vi "fissionReactorLogicAdapter.vi"(7 "Peripheral":string, 9 "State":T1={"Burn Rate"=0.0, "Formed"=FALSE, "Reactor Build Properties"={"Fuel Rods"=0, "Control Rods"=0, "Volume (m³)"=0, "Fuel Surface Area (m²)"=0, "Cooled Coolant Tank (mB)"=0, "Fuel Capacity (mB)"=0, "Heat Capacity (J/K)"=0.0, "Max Burn Rate"=0, "Max Heating Rate (mB/t)"=0, "Boil Efficiency"=0.0, "Coolant Type"=enum."Water", "Heated Coolant Tank (mB)"=0}, "Fission Reactor Build Specifications"={"Length (m)"=3, "Width (m)"=3, "Height (m)"=4, "Coolant Type"=enum."Water"}} {"Fission Reactor Build Specifications"."Height (m)" min=4 max=18 step=1; "Fission Reactor Build Specifications"."Width (m)" min=3 max=18 step=1; "Fission Reactor Build Specifications"."Length (m)" min=3 max=18 step=1; "Reactor Build Properties"."Boil Efficiency" format="%#.6g"}, 10 "Function":string, 11 "Mode":enum16{"Publish", "Read", "Handle", "Command"}(ring)) -> (3 "JSON":string)   [LabVIEW 2026]
uses:
  fissionReactor_State.ctl
  Fission Reactor Build Properties.ctl
  Fission Reactor Build Specifications.ctl
  Reactor Functions.ctl
  fissionReactor_Controls.ctl
  JSONBoolean.vi
  JSONInt64.vi
  JSONDouble.vi
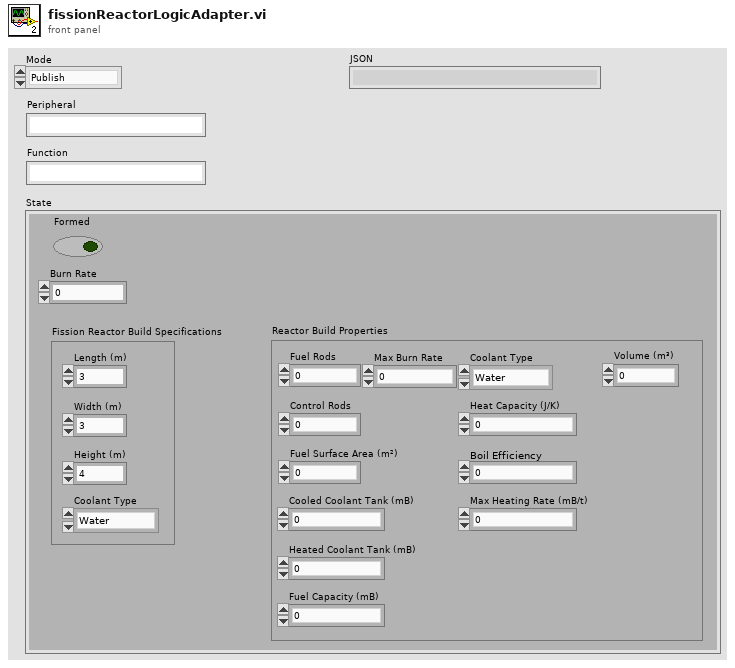
[diagram p1: front panel]
types:
  T1 = typedef "fissionReactor_State.ctl" = cluster{"Burn Rate":dbl, "Formed":bool, "Reactor Build Properties":T2, "Fission Reactor Build Specifications":T3}
  T2 = typedef "Fission Reactor Build Properties.ctl" = cluster{"Fuel Rods":i32, "Control Rods":i32, "Volume (m³)":i32, "Fuel Surface Area (m²)":i32, "Cooled Coolant Tank (mB)":i32, "Fuel Capacity (mB)":i64, "Heat Capacity (J/K)":dbl, "Max Burn Rate":i64, "Max Heating Rate (mB/t)":i64, "Boil Efficiency":dbl, "Coolant Type":enum16{"Water", "Sodium"}, "Heated Coolant Tank (mB)":i64}
  T3 = typedef "Fission Reactor Build Specifications.ctl" = cluster{"Length (m)":i32, "Width (m)":i32, "Height (m)":i32, "Coolant Type":enum16{"Water", "Sodium"}}
  T4 = typedef "fissionReactor_Controls.ctl" = cluster{"Burn Rate":dbl}
  T5 = typedef "Reactor Functions.ctl" = enum16{"isFormed", "getLength", "getWidth", "getHeight", "getMinPos", "getMaxPos", "activate", "getActualBurnRate", "getBoilEfficiency", "getBurnRate", "getCoolant", "getCoolantCapacity", "getCoolantFilledPercentage", "getCoolantNeeded", "getDamagePercent"}
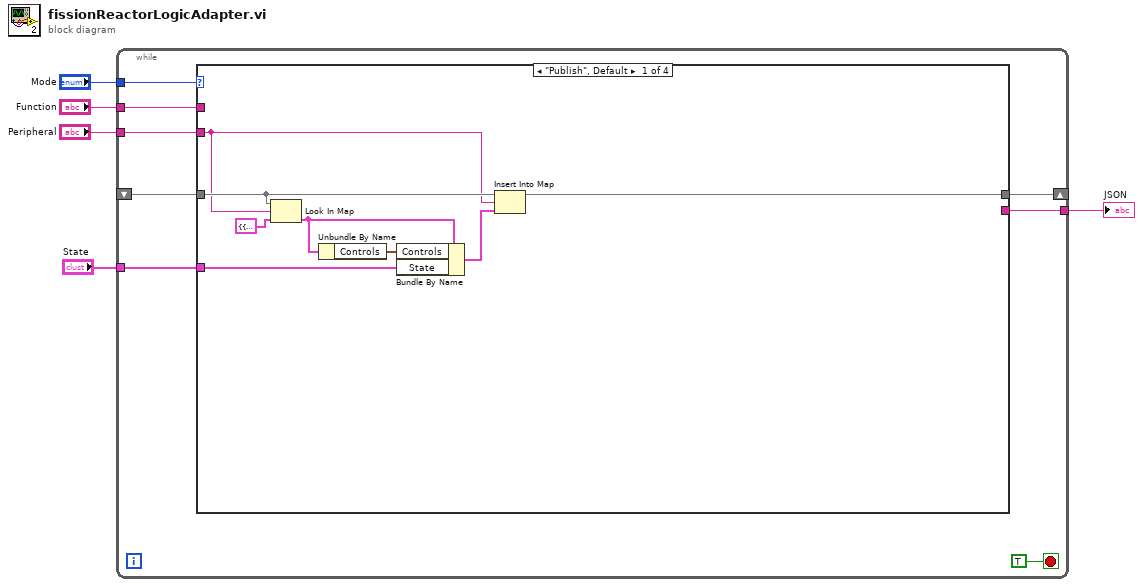
[diagram p0: block diagram]
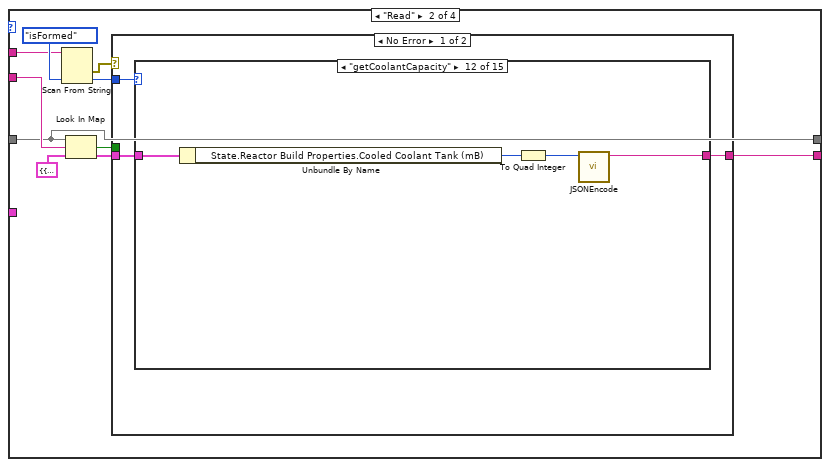
[diagram p2: hidden frame]
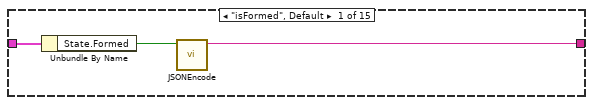
[diagram p3: hidden frame]
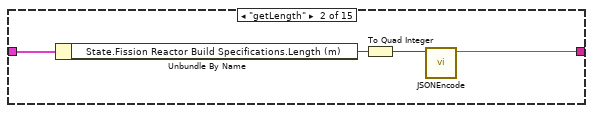
[diagram p4: hidden frame]
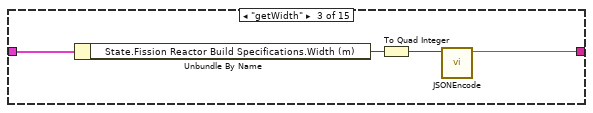
[diagram p5: hidden frame]
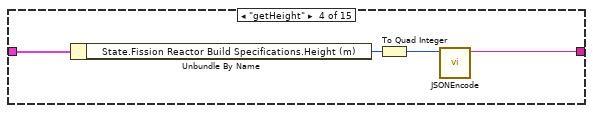
[diagram p6: hidden frame]
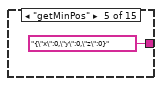
[diagram p7: hidden frame]
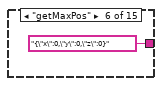
[diagram p8: hidden frame]
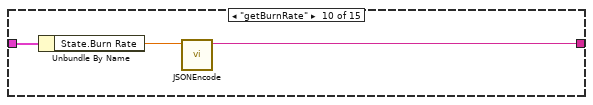
[diagram p12: hidden frame]
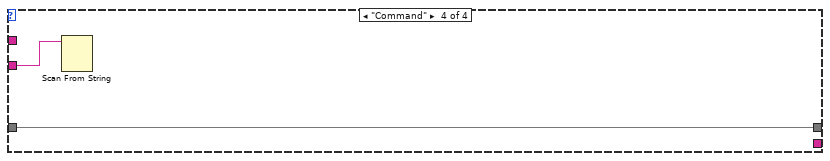
[diagram p19: hidden frame]
diagram:
  n1 = while {
    tunnel: "Mode" -> [w12]
    tunnel: "Peripheral" -> [w11]
    shift-right: [w8] -> _
    shift-left: _ -> [w10]
    tunnel: "State" -> [w9]
    tunnel: "Function" -> [w7]
    tunnel: [w6] -> w1
    stop <- TRUE stop-if-true
    n2 = case shown="\"Publish\", Default" w12 {
      tunnel: w11 -> [w15 w25 _ w61]
      tunnel: w10 -> [w16 w22 w59 w60]
      tunnel: w9 -> [w19 _ _ _]
      tunnel: [w14 w22 w59 w60] -> w8
      tunnel: w7 -> [_ w28 _ _]
      tunnel: [_ w23 _ _] -> w6
      frame "Publish", Default {
        n3 = Look In Map(map=w16, key=w15, default value=cluster{"Controls":T4, "State":T1} {"Controls"={"Burn Rate"=0.0}, "State"={"Burn Rate"=0.0, "Formed"=FALSE, "Reactor Build Properties"={"Fuel Rods"=0, "Control Rods"=0, "Volume (m³)"=0, "Fuel Surface Area (m²)"=0, "Cooled Coolant Tank (mB)"=0, "Fuel Capacity (mB)"=0, "Heat Capacity (J/K)"=0.0, "Max Burn Rate"=0, "Max Heating Rate (mB/t)"=0, "Boil Efficiency"=0.0, "Coolant Type"=enum."Water", "Heated Coolant Tank (mB)"=0}, "Fission Reactor Build Specifications"={"Length (m)"=3, "Width (m)"=3, "Height (m)"=4, "Coolant Type"=enum."Water"}}} ("Fission Reactor Data")) -> (value=w18:cluster{"Controls":T4, "State":T1})  [unwired: 1 out]
        n4 = Unbundle By Name(w18) -> ("Controls"=w21:T4)
        n5 = Bundle By Name(cluster=w18, "Controls"=w21, "State"=w19) -> (w17:cluster{"Controls":T4, "State":T1})
        n6 = Insert Into Map(map in=w16, key=w15, value=w17) -> (map out=w14:map{string, cluster{"Controls":T4, "State":T1}})  [unwired: 2 out]
      }
      frame "Read" {
        n7 = Scan From String(input string=w28, default 1=Reactor_Functions."isFormed" ("Reactor Function")) -> (error out=w31:errorcluster, output 1=w30:T5)  [unwired: 3 in, 2 out]
        n8 = Look In Map(map=w22, key=w25, default value=cluster{"Controls":T4, "State":T1} {"Controls"={"Burn Rate"=0.0}, "State"={"Burn Rate"=0.0, "Formed"=FALSE, "Reactor Build Properties"={"Fuel Rods"=0, "Control Rods"=0, "Volume (m³)"=0, "Fuel Surface Area (m²)"=0, "Cooled Coolant Tank (mB)"=0, "Fuel Capacity (mB)"=0, "Heat Capacity (J/K)"=0.0, "Max Burn Rate"=0, "Max Heating Rate (mB/t)"=0, "Boil Efficiency"=0.0, "Coolant Type"=enum."Water", "Heated Coolant Tank (mB)"=0}, "Fission Reactor Build Specifications"={"Length (m)"=3, "Width (m)"=3, "Height (m)"=4, "Coolant Type"=enum."Water"}}} ("Fission Reactor Data")) -> (key not found?=w24:bool, value=w26:cluster{"Controls":T4, "State":T1})
        n9 = case shown="No Error" w31 {
          tunnel: w30 -> [w34 _]
          tunnel: w26 -> [w33 _]
          tunnel: w24 -> [_ _]
          tunnel: [w32 _] -> w23
          frame No Error {
            n10 = case shown="\"getCoolantCapacity\"" w34 {
              tunnel: w33 -> [w37 w41 w43 w47 _ _ _ _ _ w54 _ w56 _ _ _]
              tunnel: [w36 w39 w42 w46 "{\"x\":0,\"y\":0,\"z\":0}" ("JSON string") "{\"x\":0,\"y\":0,\"z\":0}" ("JSON string") _ _ _ w52 _ w55 _ _ _] -> w32
              frame "isFormed", Default {
                n11 = Unbundle By Name(w37) -> ("State.Formed"=w35:bool)
                n12 = call-poly "JSONEncode.vi"("return"=w35) -> ("JSON string"=w36:string)  [unwired: 8 in]
              }
              frame "getLength" {
                n13 = Unbundle By Name(w41) -> ("State.Fission Reactor Build Specifications.Length (m)"=w40:i32)
                n14 = To Quad Integer(1:w40) -> (0:w38:i64)
                n15 = call-poly "JSONEncode.vi"("return"=w38) -> ("JSON string"=w39:string)  [unwired: 8 in]
              }
              frame "getWidth" {
                n16 = Unbundle By Name(w43) -> ("State.Fission Reactor Build Specifications.Width (m)"=w45:i32)
                n17 = To Quad Integer(1:w45) -> (0:w44:i64)
                n18 = call-poly "JSONEncode.vi"("return"=w44) -> ("JSON string"=w42:string)  [unwired: 8 in]
              }
              frame "getHeight" {
                n19 = Unbundle By Name(w47) -> ("State.Fission Reactor Build Specifications.Height (m)"=w49:i32)
                n20 = To Quad Integer(1:w49) -> (0:w48:i64)
                n21 = call-poly "JSONEncode.vi"("return"=w48) -> ("JSON string"=w46:string)  [unwired: 8 in]
              }
              frame "getMinPos" {
              }
              frame "getMaxPos" {
              }
              frame "activate" {
              }
              frame "getActualBurnRate" {
              }
              frame "getBoilEfficiency" {
              }
              frame "getBurnRate" {
                n22 = Unbundle By Name(w54) -> ("State.Burn Rate"=w53:dbl)
                n23 = call-poly "JSONEncode.vi"("return"=w53) -> ("JSON string"=w52:string)  [unwired: 8 in]
              }
              frame "getCoolant" {
              }
              frame "getCoolantCapacity" {
                n24 = Unbundle By Name(w56) -> ("State.Reactor Build Properties.Cooled Coolant Tank (mB)"=w58:i32)
                n25 = To Quad Integer(1:w58) -> (0:w57:i64)
                n26 = call-poly "JSONEncode.vi"("return"=w57) -> ("JSON string"=w55:string)  [unwired: 8 in]
              }
              frame "getCoolantFilledPercentage" {
              }
              frame "getCoolantNeeded" {
              }
              frame "getDamagePercent" {
              }
            }
          }
          frame Error {
          }
        }
      }
      frame "Handle" {
      }
      frame "Command" {
        n27 = Scan From String(input string=w61) -> ()  [unwired: 5 in, 3 out]
      }
    }
  }
  "JSON" <- w1
